vi "Create All Custom Chars.vi"(8 "error in (no error)":errorcluster, 9 "Custom Chars":T2, 10 "Session In":refnum<class "Session.lvclass">, 11 "Grove I2C LCD in":refnum<class "Grove I2C LCD.lvclass">) -> (0 "error out":errorcluster, 2 "Session Out":refnum<class "Session.lvclass">, 3 "Grove I2C LCD out":refnum<class "Grove I2C LCD.lvclass">)   [LabVIEW 2020, in "CTI-Peripheral.lvlib" / "Grove I2C LCD.lvclass"]
uses:
  Grove I2C LCD.lvclass
  CTI/Session/Session.lvclass
  CTI-Visa-DeviceLib/LCD-I2C/Custom Char.ctl
  CTI-Visa-DeviceLib/LCD-I2C/LCD-I2C.lvclass
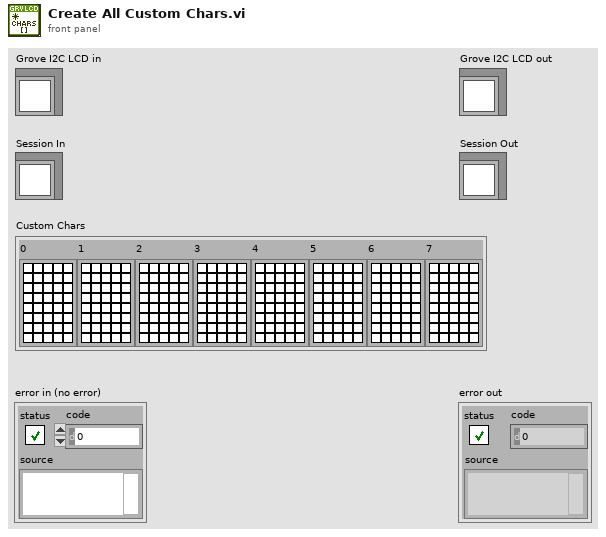
[diagram p1: front panel]
types:
  T1 = typedef "CTI-Visa-DeviceLib.lvlib/LCD-I2C.lvclass/Custom Char.ctl" = bool[][]
  T2 = cluster{"0":T1, "1":T1, "2":T1, "3":T1, "4":T1, "5":T1, "6":T1, "7":T1}
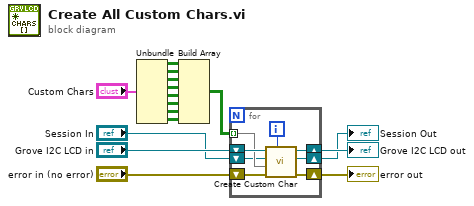
[diagram p0: block diagram]
diagram:
  n1 = Unbundle("Custom Chars") -> ("0"=w14:T1, "1"=w13:T1, "2"=w12:T1, "3"=w11:T1, "4"=w10:T1, "5"=w9:T1, "6"=w8:T1, "7"=w7:T1)
  n2 = Build Array(w14, w13, w12, w11, w10, w9, w8, w7) -> (w3:bool[][][])
  n3 = for {
    shift-right: [w23] -> w6
    shift-left: "error in (no error)" -> [w24]
    shift-right: [w21] -> w4
    shift-left: "Grove I2C LCD in" -> [w22]
    tunnel: w3 -> [w19] mode=indexing
    shift-right: [w17] -> w1
    shift-left: "Session In" -> [w18]
    i -> [w20]
    n4 = call-dynamic "Create Custom Char.vi"("Char #"=w20, "error in (no error)"=w24, "Char"=w19, "Session In"=w18, "Character LCD in"=w22) -> ("error out"=w23:errorcluster, "Session Out"=w17:refnum<class "Session.lvclass">, "Character LCD out"=w21:refnum<class "Grove I2C LCD.lvclass">)  [unwired: 4 in]
  }
  "error out" <- w6
  "Grove I2C LCD out" <- w4
  "Session Out" <- w1
